vi "92429239ModulePresent.vi"(11 "all dynamic modules":string[](array[string])) -> (1 "9239 present":bool, 2 "9242 present":bool, 3 "9242&9239 present":bool)   [LabVIEW 2017, in "McsaFpgaBitfileManager.lvlib"]
uses:
  <vilib>/addons/InsightCM/Devices/Shared/Mcsa/McsaFpgaBitfileManager/McsaFpgaBitfileManager.lvlib
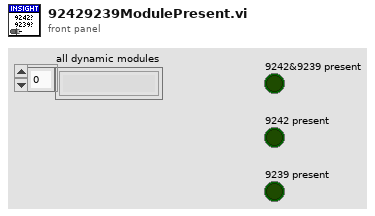
[diagram p1: front panel]
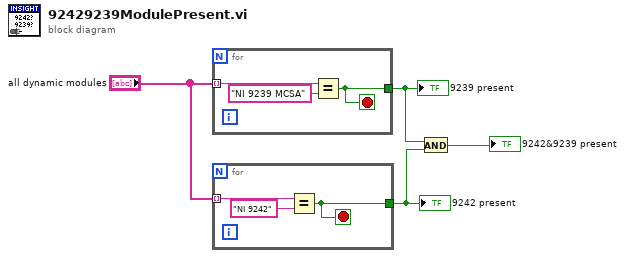
[diagram p0: block diagram]
diagram:
  n1 = for {
    tunnel: "all dynamic modules" -> [w7] mode=indexing
    tunnel: [w5] -> w3
    stop <- w5 stop-if-true
    n2 = Equal?(x=w7, y="NI 9239 MCSA") -> (x = y?=w5:bool)
  }
  "9239 present" <- w3
  n3 = for {
    tunnel: "all dynamic modules" -> [w10] mode=indexing
    tunnel: [w8] -> w2
    stop <- w8 stop-if-true
    n4 = Equal?(x=w10, y="NI 9242") -> (x = y?=w8:bool)
  }
  "9242 present" <- w2
  n5 = And(x=w3, y=w2) -> (x .and. y?=→"9242&9239 present":bool)
